vi "Stop RFSG Check.vi"(8 "error in (no error)":errorcluster, 11 "rfsg queue":refnum<queue>) -> (0 "error out":errorcluster, 3 "stop?":bool)   [LabVIEW 2021]
uses:
  Messaging/RFSG Message.ctl
  RFSG Configuration.ctl
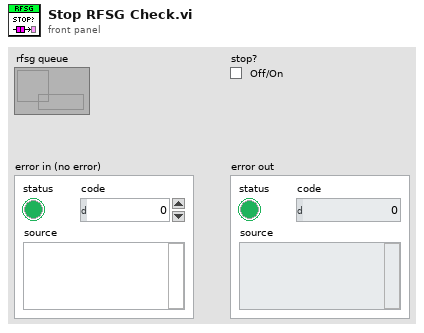
[diagram p1: front panel]
types:
  T1 = typedef "RFSG Message.ctl" = enum16{"Initialize RF", "Run RF", "Stop RF", "Exit"}
  T2 = typedef "RFSG Configuration.ctl" = cluster{"rfsg ref":refnum<k15>, "freq off":i32, "wfm type":u16, "cent freq":dbl, "iq rate":dbl, "power":dbl, "msg":T1}
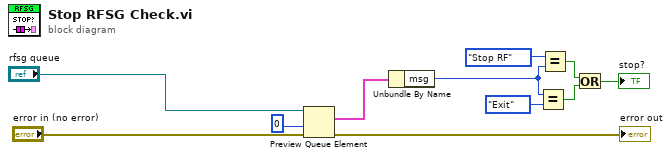
[diagram p0: block diagram]
diagram:
  n1 = Preview Queue Element(queue="rfsg queue", timeout in ms (-1)=0, error in (no error)="error in (no error)") -> (element=w11:T2, error out=→"error out":errorcluster)  [unwired: 2 out]
  n2 = Unbundle By Name(w11) -> ("msg"=w4:T1)
  n3 = Equal?(x=w4, y=RFSG_Message."Exit") -> (x = y?=w3:bool)
  n4 = Equal?(x=RFSG_Message."Stop RF" ("y"), y=w4) -> (x = y?=w2:bool)
  n5 = Or(x=w2, y=w3) -> (x .or. y?=→"stop?":bool)
